vi "startMission.vi"(8 "error in (no error)":errorcluster, 11 "StationKeeping in":refnum<class "StationKeeping.lvclass">) -> (0 "error out":errorcluster, 3 "StationKeeping out":refnum<class "StationKeeping.lvclass">)   [LabVIEW 2011, in "StationKeeping.lvclass"]
doc: "Starts the stationKeeping mission. This is different from initializing, in that it has a time sensitive value in it, so it shouldn't be called until we are ready to start the timer. If it is, we use the reset timer method to make sure our timer is correct."
uses:
  StationKeeping.lvclass
  StationKeeping.lvclass/StationKeeping.ctl
  GenericMission/GenericMission.lvclass
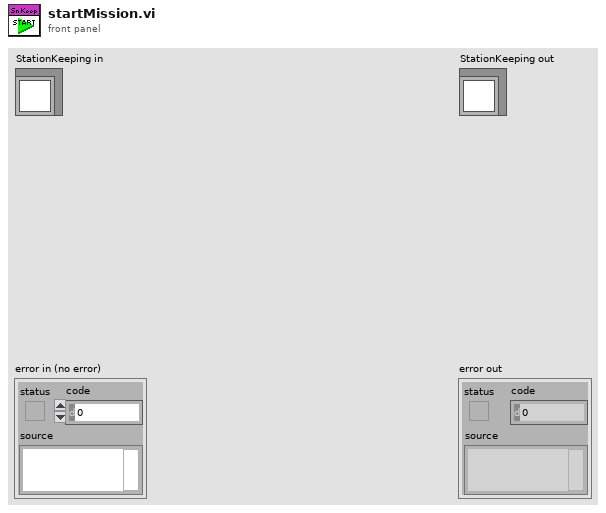
[diagram p1: front panel]
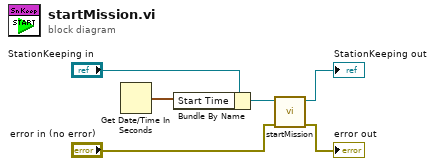
[diagram p0: block diagram]
diagram:
  n1 = Get Date/Time In Seconds() -> (seconds since 1Jan1904=w5:timestamp)
  n2 = Bundle By Name(cluster="StationKeeping in", "Start Time"=w5) -> (w4:refnum<class "StationKeeping.lvclass">)
  n3 = call-parent "startMission.vi"("error in (no error)"="error in (no error)", "GenericMission in"=w4) -> ("error out"=→"error out":errorcluster, "GenericMission out"=→"StationKeeping out":refnum<class "StationKeeping.lvclass">)  [unwired: 8 in]
